vi "CVT2LoadTags.vi"() -> (3 "Unit Test Framework Results":T1)   [LabVIEW 2013, in "UnitTests.lvlib"]
uses:
  UnitTests.lvlib
  <vilib>/utf/common/utf_test_result_troll.ctl
  <vilib>/utf/common/utf_test_result.ctl
  <vilib>/utf/common/utf_test_result_failure.ctl
  <vilib>/utf/common/utf_test_comparison_operators.ctl
  <vilib>/utf/common/utf_vi_tag.ctl
  <vilib>/NI/Current Value Table/DataTypes/Double_Read Index.vi
  <vilib>/NI/Current Value Table/Memory Block.vi
  <vilib>/NI/Current Value Table/DataTypes/Double_Memory Block.vi
  <vilib>/utf/NI_UnitTestFramework.lvlib
  <vilib>/NI/Current Value Table/Current Value Table.lvlib
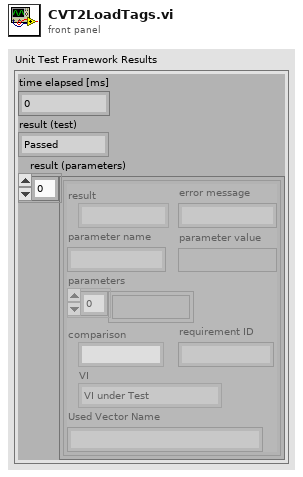
[diagram p1: front panel]
types:
  T1 = typedef "NI_UnitTestFramework.lvlib/utf_test_result_troll.ctl" = cluster{"time elapsed [ms]":u32, "result (test)":T2, "result (parameters)":T3[]}
  T2 = typedef "NI_UnitTestFramework.lvlib/utf_test_result.ctl" = enum16{"Passed", "Failed", "Error", "Skipped", "Not Processed"}
  T3 = typedef "NI_UnitTestFramework.lvlib/utf_test_result_failure.ctl" = cluster{"result":T2, "error message":string, "parameter name":string, "parameter value":variant, "parameters":variant[], "comparison":T4, "requirement ID":string, "VI":T5, "Used Vector Name":string}
  T4 = typedef "NI_UnitTestFramework.lvlib/utf_test_comparison_operators.ctl" = enum16{"=", "!=", ">", ">=", "<", "<=", "range", "symmetric tolerance", "asymmetric tolerance", "string contains", "string not contain", "array size", "string length", "array range", "by element", "array range (limit array)", "user-defined", "array contains", "array not contain", "vector length", "= (elm)", "!= (elm)", "= (case insensitive)", "!= (case insensitive)"}
  T5 = typedef "NI_UnitTestFramework.lvlib/utf_vi_tag.ctl" = enum16{"Setup VI", "VI under Test", "Teardown VI"}
  T6 = typedef "Current Value Table.lvlib/File Format.ctl" = cluster{"Tags":T7[], "Group Listings":T9[]}
  T7 = typedef "Current Value Table.lvlib/Single Tag.ctl" = cluster{"Data Type":T8, "Name":string, "Value":string, "Description":string}
  T8 = typedef "Current Value Table.lvlib/Data Types.ctl" = enum16{"Double", "Single", "I64", "I32", "I16", "I8", "U64", "U32", "U16", "U8", "String", "Boolean", "Array of U8", "Array of U16", "Array of U32", "Array of U64", "Array of I64", "Array of I32", "Array of I16", "Array of I8", "Array of Double", "Array of Single", "Array of Boolean", "Array of String"}
  T9 = typedef "Current Value Table.lvlib/Tag Grouping set.ctl" = cluster{"Group":string, "Tag Names":string[]}
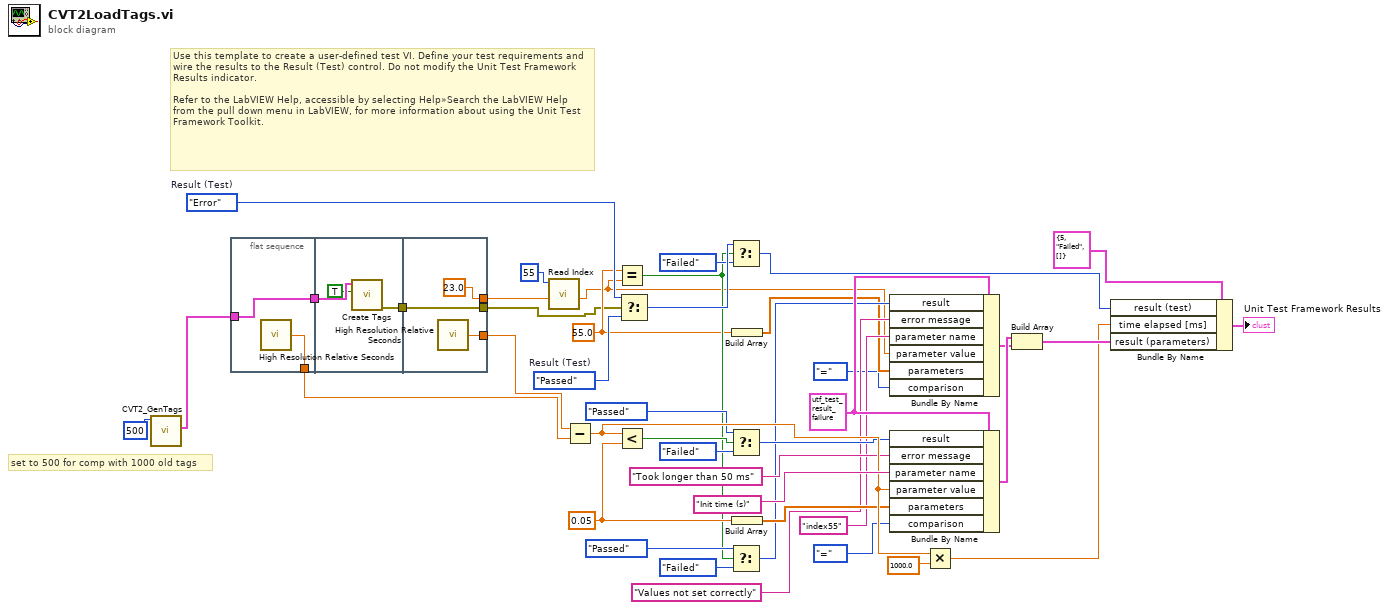
[diagram p0: block diagram]
diagram:
  w9 = 55.0 ("Index")
  w24 = 0.05 ("y")
  w17 = T3 {"result"=enum."Passed", "error message"="", "parameter name"="", "parameter value"=variant, "parameters"=[], "comparison"=enum."=", "requirement ID"="", "VI"=enum."Setup VI", "Used Vector Name"=""} ("Unit Test Framework - result (parameters)")
  w37 = utf_test_result."Error"  # Result (Test)
  w36 = utf_test_result."Passed"  # Result (Test)
  # "set to 500 for comp with 1000 old tags"
  # "Use this template to create a user-defined test VI. Define your test requirements and wire the results to the Result (Test) control. Do not modify the Unit Test Framework Results indicator. \n\nRefer to the LabVIEW Help, accessible by selecting Help»Search the LabVIEW Help from the pull down menu in LabVIEW, for more information about using the Unit Test Framework Toolkit."
  n1 = call "CVT2_GenTags.vi"("Tags per type"=500) -> ("Init data"=w6:T6)  [unwired: 7 in, 3 out]
  n2 = flat-sequence {
    tunnel: [w44] -> w39
    tunnel: w6 -> [w43]
    tunnel: [w43] -> w5
    tunnel: [w47] -> w31
    tunnel: w5 -> [w46]
    tunnel: [w50] -> w40
    tunnel: [w49] -> w3
    tunnel: w31 -> [w49]
    tunnel: [23.0 ("Default")] -> w1
    frame #0 {
      n3 = call <vilib>:"High Resolution Relative Seconds.vi"() -> ("relative seconds"=w44:dbl)
    }
    frame #1 {
      n4 = call <vilib>:"Create Tags.vi"("Clear Table? (F)"=TRUE, "CVT Tags to Create"=w46) -> ("error out"=w47:errorcluster)  [unwired: 9 in]
    }
    frame #2 {
      n5 = call <vilib>:"High Resolution Relative Seconds.vi"() -> ("relative seconds"=w50:dbl)
    }
  }
  n6 = call-poly <vilib>:"Read Index.vi"("Default"=w1, "Index"=55) -> ("Value"=w2:dbl)  [unwired: 9 in]
  n7 = Subtract(x=w40, y=w39) -> (x-y=w30:dbl)
  n8 = Equal?(x=w9, y=w2) -> (x = y?=w13:bool)
  n9 = Less?(x=w30, y=w24) -> (x < y?=w23:bool)
  n10 = Select(t=w37, s=w3, f=w36) -> (s? t:f=w21:T2)
  n11 = Select(t=w21, s=w13, f=utf_test_result."Failed") -> (s? t:f=w19:T2)
  n12 = Select(t=utf_test_result."Passed" ("result"), s=w23, f=utf_test_result."Failed" ("result")) -> (s? t:f=w29:T2)
  n13 = Select(t=utf_test_result."Passed" ("result"), s=w13, f=utf_test_result."Failed" ("result")) -> (s? t:f=w14:T2)
  n14 = Build Array(w9) -> (w10:dbl[])
  n15 = Build Array(w24) -> (w25:dbl[])
  n16 = Bundle By Name(cluster=w17, "result"=w14, "error message"="Values not set correctly", "parameter name"="index55", "parameter value"=w2, "parameters"=w10, "comparison"=utf_test_comparison_operators."=") -> (w18:T3)
  n17 = Bundle By Name(cluster=w17, "result"=w29, "error message"="Took longer than 50 ms", "parameter name"="Init time (s)", "parameter value"=w30, "parameters"=w25, "comparison"=utf_test_comparison_operators."=") -> (w35:T3)
  n18 = Multiply(x=w30, y=1000.0) -> (x*y=w32:dbl)
  n19 = Build Array(w35, w18) -> (w34:T3[])
  n20 = Bundle By Name(cluster=T1 {"time elapsed [ms]"=5, "result (test)"=enum."Failed", "result (parameters)"=[]} ("Unit Test Framework - Result"), "result (test)"=w19, "time elapsed [ms]"=w32, "result (parameters)"=w34) -> (→"Unit Test Framework Results":T1)
